vi "Launcher.vi"() -> ()   [LabVIEW 2021]
uses:
  Model/Model.lvlib
  <vilib>/DQMH Consortium/Lumos API/Libraries/SDV API/SDV API.lvlib
panel:
  out "Tracing?":bool
  in  "Tracing En/Dis":bool
  in  "Get Status":bool
  in  "Add Divider":bool
  in  "Exit":bool
  in  "Stop":bool
  in  "Start":bool
  # "Application \nLauncher"
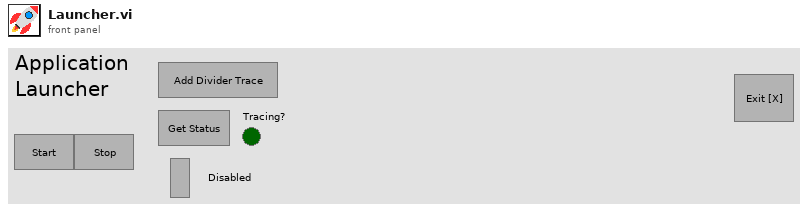
[diagram p1: front panel]
types:
  T1 = typedef "Model.lvlib/Broadcast Events--cluster.ctl" = cluster{"Module Did Init":refnum<user-event>, "Status Updated":refnum<user-event>, "Error Reported":refnum<user-event>, "Module Did Stop":refnum<user-event>, "Update Module Execution Status":refnum<user-event>}
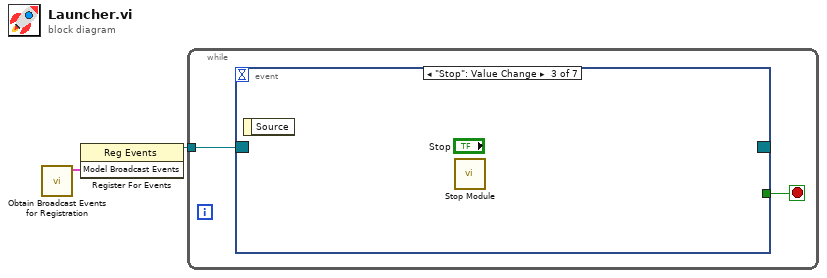
[diagram p0: block diagram]
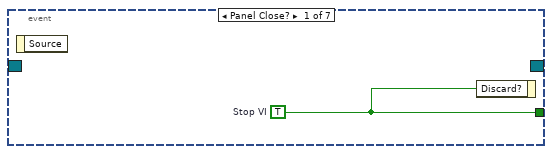
[diagram p2: hidden frame]
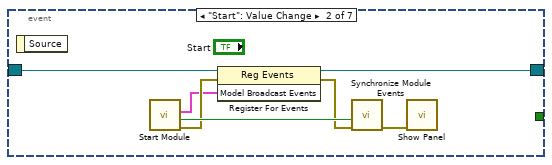
[diagram p3: hidden frame]
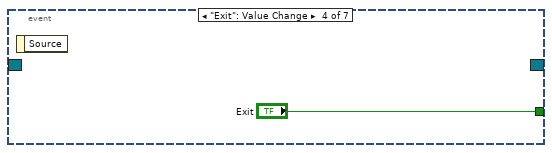
[diagram p4: hidden frame]
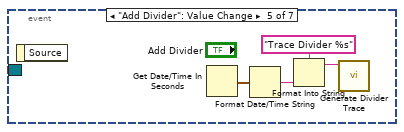
[diagram p5: hidden frame]
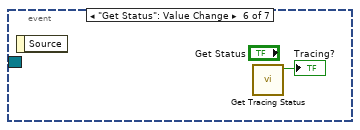
[diagram p6: hidden frame]
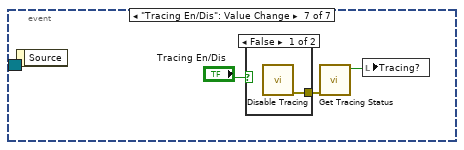
[diagram p7: hidden frame]
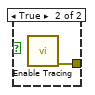
[diagram p8: hidden frame]
diagram:
  n1 = call "Obtain Broadcast Events for Registration.vi"() -> ("Model Broadcast Events"=w1:T1)  [unwired: 9 in, 2 out]
  n2 = register-events(w1) -> (reference out=w2:refnum<event-registration>)  [unwired: 2 in, 1 out]
  n3 = while {
    tunnel: w2 -> [w3]
    stop <- w4 stop-if-true
    n4 = event shown="[2] \"Stop\": Value Change" {
      selector: w3 -> [_ w7 _ _ _ _ _]
      dyn-events: [_ w6 _ _ _ _ _] -> _
      timeout: _ -> [_ _ _ _ _ _ _]
      tunnel: [w5 _ _ "Exit" _ _ _] -> w4
      event Panel Close? {
        w5 = TRUE  # Stop VI
        n5 = event-data() -> ()  [unwired: 1 in, 1 out]
        n6 = event-data("Discard?"=w5) -> ()  [unwired: 1 in, 1 out]
      }
      event "Start": Value Change {
        n7 = event-data() -> ()  [unwired: 1 in, 1 out]
        n8 = call "Start Module.vi"() -> ("error out"=w9:errorcluster, "Wait for Event Sync?"=w11:bool, "Model Broadcast Events"=w8:T1)  [unwired: 8 in, 1 out]
        n9 = register-events(reference=w7, error in=w9, w8) -> (reference out=w6:refnum<event-registration>, error out=w10:errorcluster)
        n10 = call "Synchronize Module Events.vi"("error in (no error)"=w10, "Wait for Event Sync?"=w11) -> ("error out"=w12:errorcluster)  [unwired: 9 in]
        n11 = call "Show Panel.vi"("error in (no error)"=w12) -> ()  [unwired: 10 in, 1 out]
      }
      event "Stop": Value Change {
        n12 = event-data() -> ()  [unwired: 1 in, 1 out]
        n13 = call "Stop Module.vi"() -> ()  [unwired: 11 in, 1 out]
      }
      event "Exit": Value Change {
        n14 = event-data() -> ()  [unwired: 1 in, 1 out]
      }
      event "Add Divider": Value Change {
        n15 = event-data() -> ()  [unwired: 1 in, 1 out]
        n16 = Get Date/Time In Seconds() -> (seconds since 1Jan1904=w17:timestamp)
        n17 = Format Date/Time String(seconds (now)=w17) -> (date/time string=w16:string)  [unwired: 2 in]
        n18 = Format Into String(format string="Trace Divider %s", w16) -> (resulting string=w14:string)  [unwired: 2 in, 1 out]
        n19 = call <vilib>:"Generate Divider Trace.vi"("Message"=w14) -> ()  [unwired: 10 in, 1 out]
      }
      event "Get Status": Value Change {
        n20 = event-data() -> ()  [unwired: 1 in, 1 out]
        n21 = call <vilib>:"Get Tracing Status.vi"() -> ("Tracing Enabled?"=→"Tracing?":bool)  [unwired: 10 in, 1 out]
      }
      event "Tracing En/Dis": Value Change {
        n22 = event-data() -> ()  [unwired: 1 in, 1 out]
        n23 = case shown="False" "Tracing En/Dis" {
          tunnel: [w22 w23] -> w21
          frame False {
            n24 = call <vilib>:"Disable Tracing.vi"() -> ("error out"=w22:errorcluster)  [unwired: 11 in]
          }
          frame True {
            n25 = call <vilib>:"Enable Tracing.vi"() -> ("error out"=w23:errorcluster)  [unwired: 11 in]
          }
        }
        n26 = call <vilib>:"Get Tracing Status.vi"("error in"=w21) -> ("Tracing Enabled?"=w19:bool)  [unwired: 9 in, 1 out]
        n27 = local write "Tracing?"(w19) -> ()
      }
    }
  }
